vi "add amp gain metadata.vi"(8 "error in (no error)":errorcluster, 11 "Metadata in":string[][](array[string])) -> (0 "error out":errorcluster, 3 "Metadata out":string[][](array[string]))   [LabVIEW 2013]
panel:
  in  "Continue?":bool
  in  "Amp Gain Range":string(combo)
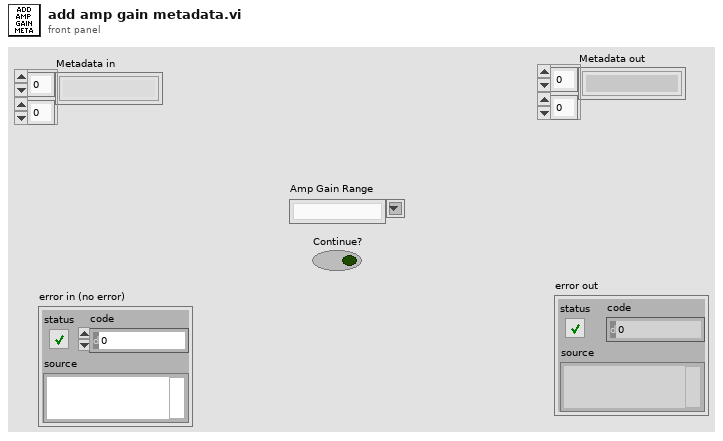
[diagram p1: front panel]
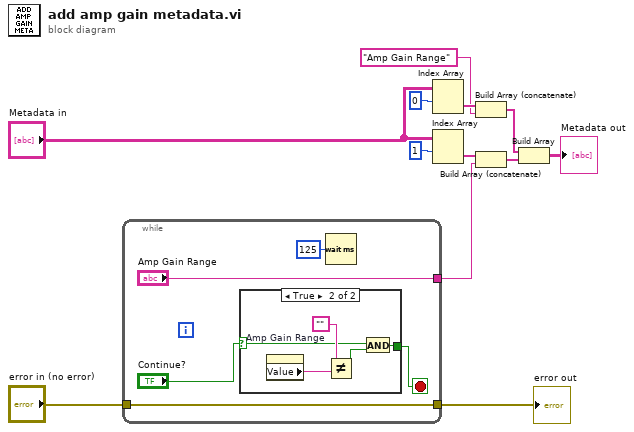
[diagram p0: block diagram]
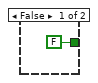
[diagram p2: hidden frame]
diagram:
  n1 = while {
    tunnel: ["Amp Gain Range"] -> w1
    tunnel: "error in (no error)" -> [w16]
    tunnel: [w16] -> w2
    stop <- w13 stop-if-true
    n2 = case shown="True" "Continue?" {
      selector: "Continue?" -> [_ w20]
      tunnel: [FALSE w19] -> w13
      frame False {
      }
      frame True {
        n3 = property on="Amp Gain Range" class="CmbBox"() -> ("Value"=w22:string)  [unwired: 2 in, 2 out]
        n4 = Not Equal?(x="", y=w22) -> (x != y?=w21:bool)
        n5 = And(x=w20, y=w21) -> (x .and. y?=w19:bool)
      }
    }
    n6 = Wait (ms)(milliseconds to wait=u32 125) -> ()  [unwired: 1 out]
  }
  "error out" <- w2
  n7 = Index Array(array="Metadata in", index (row)=0 ("index")) -> (element=w9:string[])  [unwired: 1 in]
  n8 = Index Array(array="Metadata in", index (row)=1 ("index")) -> (element=w7:string[])  [unwired: 1 in]
  n9 = Build Array (concatenate)(w9, "Amp Gain Range") -> (w6:string[])
  n10 = Build Array (concatenate)(w7, w1) -> (w5:string[])
  n11 = Build Array(w6, w5) -> (→"Metadata out":string[][])
